vi "TSC Material Color Roles--constant.vi"() -> (2 "Control Color Roles":string[](array[string]))   [LabVIEW 2021, in "Material SubVIs.lvlib"]
doc: "CONSTANT VI defines the constant value for the Control Color Roles that are shown in the right click menu and are used in color application.\n\n<b>Code Developed By:</b> +\nDaniel Coons +\nTechnology Service Corporation +\nwww.tsc.com/atcs"
uses:
  Material SubVIs.lvlib
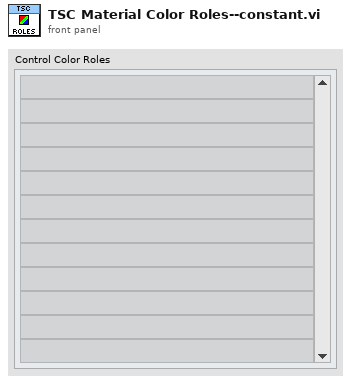
[diagram p1: front panel]
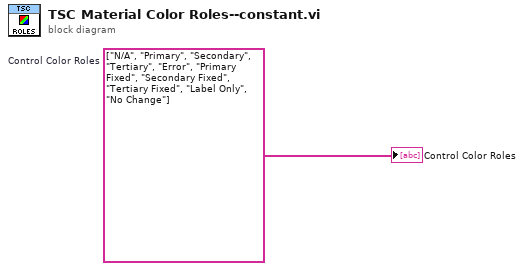
[diagram p0: block diagram]
diagram:
  w1 = string[] ["N/A", "Primary", "Secondary", "Tertiary", "Error", "Primary Fixed", "Secondary Fixed", "Tertiary Fixed", "Label Only", "No Change"]  # Control Color Roles
  "Control Color Roles" <- w1
